vi "Do.vi"(8 "error in (no error)":errorcluster, 10 "Actor in":refnum<class "Actor.lvclass">, 11 "Change Setpoint Msg":refnum<class "Change Desired Temperature Msg.lvclass">) -> (0 "error out":errorcluster, 2 "Actor out":refnum<class "Actor.lvclass">)   [LabVIEW 2012, in "Cooler UI.lvlib" / "Change Desired Temperature Msg.lvclass"]
uses:
  Change Desired Temperature Msg.lvclass
  <vilib>/ActorFramework/Actor/Actor.lvclass
  Cooler UI with Events/Cooler UI with Events.lvclass
  Change Desired Temperature Msg.lvclass/Change Desired Temperature Msg.ctl
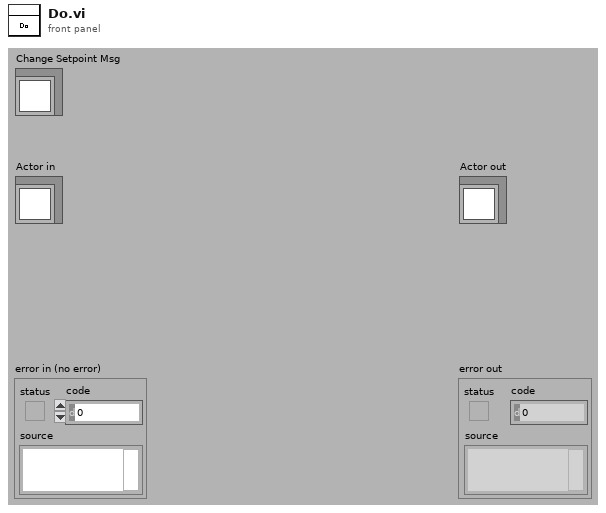
[diagram p1: front panel]
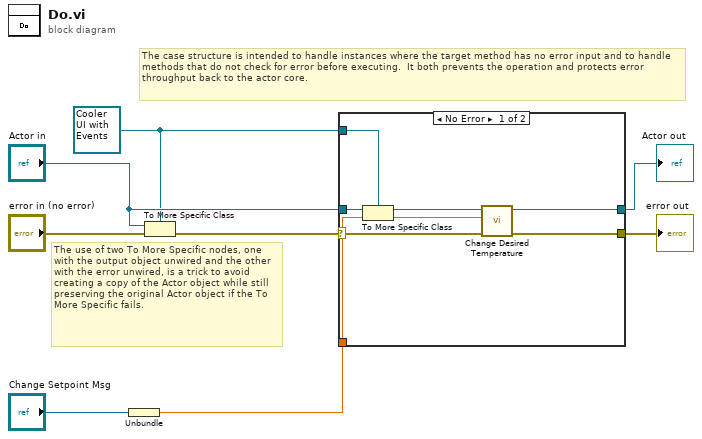
[diagram p0: block diagram]
diagram:
  w2 = refnum<class "Cooler UI with Events.lvclass"> refnum ("Actor in")
  # "The use of two To More Specific nodes, one with the output object unwired and the other with the error unwired, is a trick to avoid creating a copy of the Actor object while still preserving the original Actor object if the To More Specific fails."
  # "The case structure is intended to handle instances where the target method has no error input and to handle methods that do not check for error before executing.  It both prevents the operation and protects error throughput back to the actor core."
  n1 = Unbundle("Change Setpoint Msg") -> (w1:dbl)
  n2 = To More Specific Class(target class=w2, reference="Actor in", error in="error in (no error)") -> (error out=w6:errorcluster)  [unwired: 1 out]
  n3 = case shown="No Error" w6 {
    selector: w6 -> [w13 w17]
    tunnel: [w15 w17] -> w5
    tunnel: [w14 w16] -> w4
    tunnel: "Actor in" -> [w12 w16]
    tunnel: w2 -> [w11 _]
    tunnel: w1 -> [w9 _]
    frame No Error {
      n4 = To More Specific Class(target class=w11, reference=w12) -> (specific class reference=w10:refnum<class "Cooler UI with Events.lvclass">)  [unwired: 1 in, 1 out]
      n5 = call "Change Desired Temperature.vi"("error in (no error)"=w13, "Desired Temperature"=w9, "Cooler UI with Events in"=w10) -> ("error out"=w15:errorcluster, "Cooler UI with Events out"=w14:refnum<class "Cooler UI with Events.lvclass">)  [unwired: 7 in]
    }
    frame Error {
      # "If type check fails, pass the original object out again."
    }
  }
  "error out" <- w5
  "Actor out" <- w4
